vi "XIPIN_AXI_Protocol_Converter_2_1.vi"   [LabVIEW 2017]
doc: "The AXI Protocol Converter IP provides the facility to change the protocol of the connection between an AXI4/AXI3/AXI4-Lite master and slave. It will convert between AXI4->AXI3/AXI4-Lite, AXI3->AXI4/AXI4-Lite, AXI4-Lite->AXI4/AXI3.\n------------------------------------\n<b>Need License</b> : No\n<b>Interface</b> : AXI4"
uses:
  <vilib>/rvi/XilinxIP/XIPIN_XNode/niFpgaXIPIN.xnode
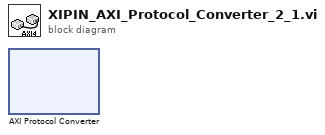
[diagram p0: block diagram]
diagram:
  n1 = xnode ("AXI Protocol Converter")() -> ()
